vi "RebuildCmdListing.vi"(3 "Numeric":dbl, 4 "Contents":string, 5 "Params":T1(array[cluster]), 6 "String in":string) -> (1 "array":string[](array[string]), 2 "String out":string)   [LabVIEW 2012]
panel:
  out "Array":dbl[](array[numeric])
  out "Contents 2":string
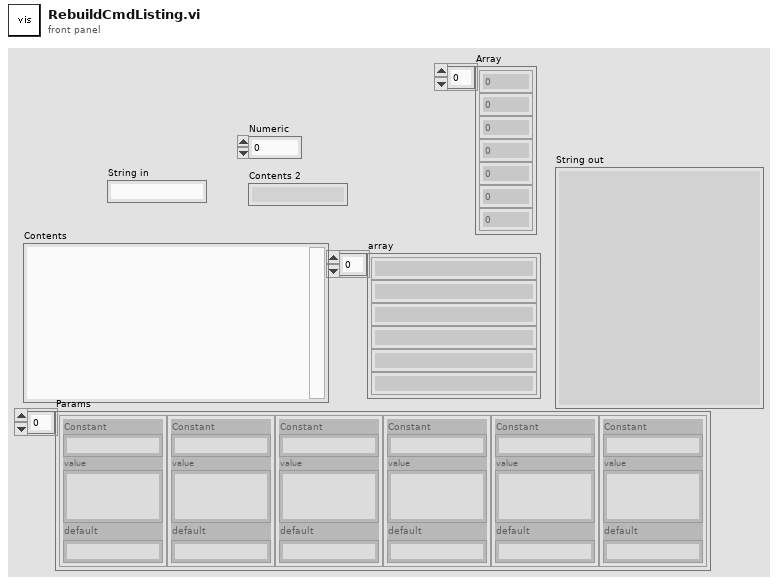
[diagram p1: front panel]
types:
  T1 = cluster{"Constant":string, "value":string, "default":string}[]
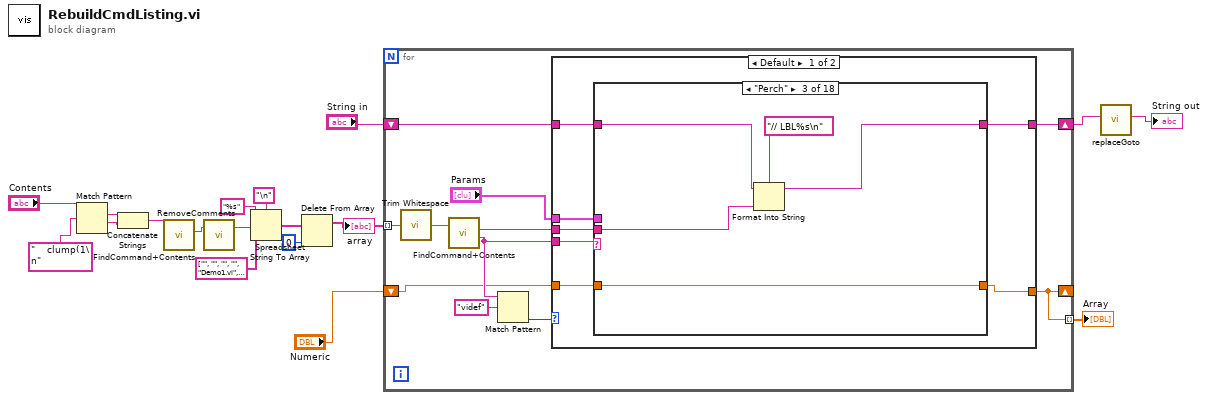
[diagram p0: block diagram]
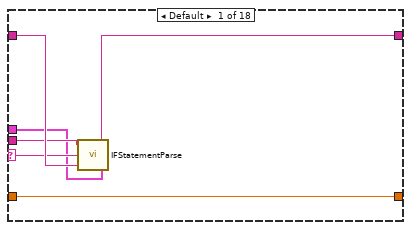
[diagram p2: hidden frame]
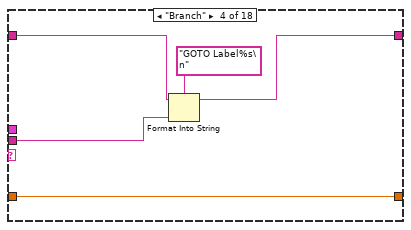
[diagram p4: hidden frame]
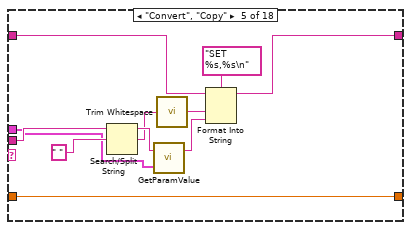
[diagram p5: hidden frame]
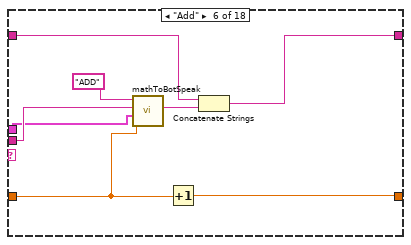
[diagram p6: hidden frame]
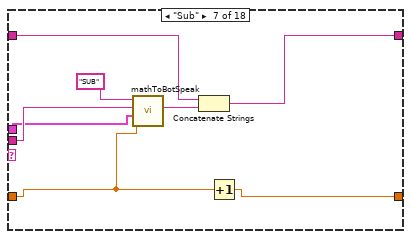
[diagram p7: hidden frame]
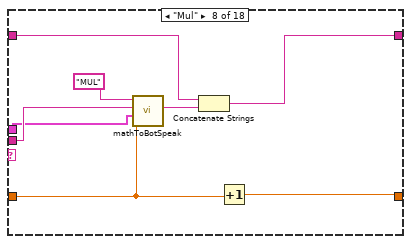
[diagram p8: hidden frame]
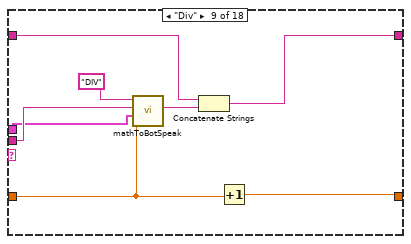
[diagram p9: hidden frame]
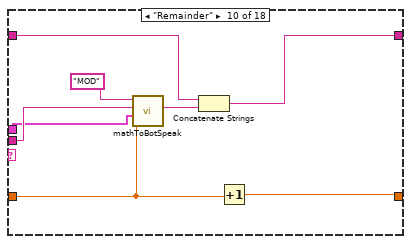
[diagram p10: hidden frame]
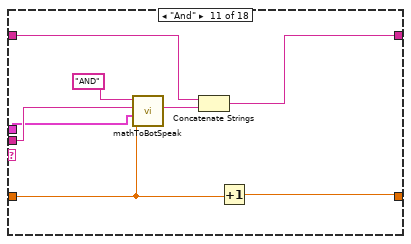
[diagram p11: hidden frame]
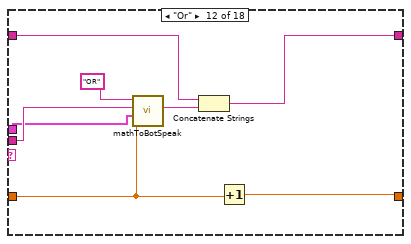
[diagram p12: hidden frame]
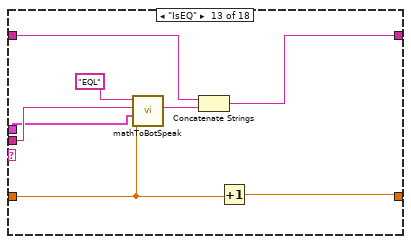
[diagram p13: hidden frame]
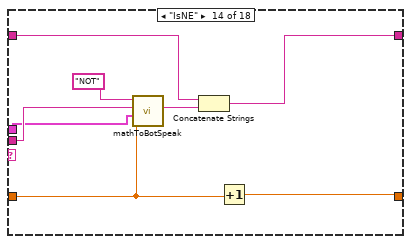
[diagram p14: hidden frame]
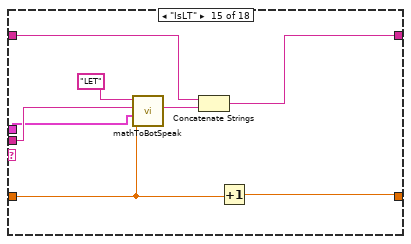
[diagram p15: hidden frame]
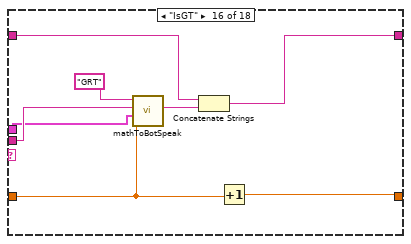
[diagram p16: hidden frame]
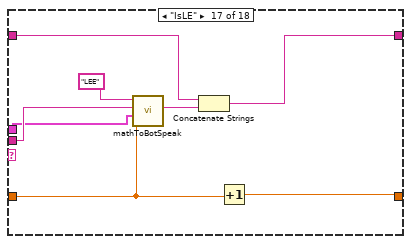
[diagram p17: hidden frame]
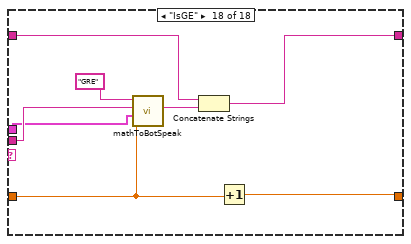
[diagram p18: hidden frame]
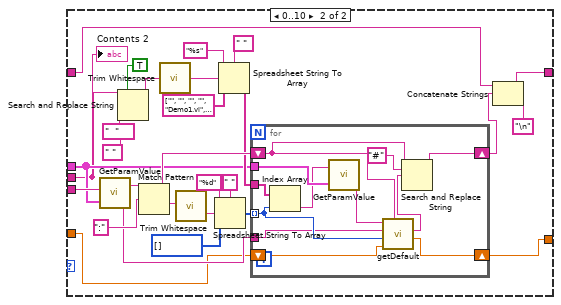
[diagram p19: hidden frame]
diagram:
  n1 = Match Pattern(string="Contents", regular expression="    clump(1\n") -> (match substring=w10:string, after substring=w11:string)  [unwired: 1 in, 2 out]
  n2 = Concatenate Strings(w10, w11) -> (w12:string)
  n3 = call <userlib>:"FindCommand+Contents.vi"("Via file in"=w12) -> ("Contents"=w13:string)  [unwired: 1 in, 3 out]
  n4 = call <userlib>:"RemoveComments.vi"("Via file in"=w13) -> ("Via file out"=w14:string)  [unwired: 2 in]
  n5 = Spreadsheet String To Array(delimiter (Tab)="\n", format string="%s", spreadsheet string=w14, array type (2D Dbl)=string[] ["", "", "", "", "Demo1.vi", "DigitalWrite.vi", "VS_Wait.vi", ""] ("Array 3")) -> (array=w17:string[])
  n6 = Delete From Array(array=w17, index=0) -> (array with subset deleted=w6:string[])  [unwired: 1 in, 1 out]
  "array" <- w6
  n7 = for {
    tunnel: w6 -> [w29] mode=indexing
    shift-right: [w26] -> w4
    shift-left: "String in" -> [w27]
    shift-right: [w19] -> _
    shift-left: "Numeric" -> [w20]
    tunnel: [w19] -> w2 mode=indexing
    n8 = call <vilib>:"Trim Whitespace.vi"("string"=w29) -> ("trimmed string"=w28:string)  [unwired: 1 in]
    n9 = call <userlib>:"FindCommand+Contents.vi"("Via file in"=w28) -> ("Contents"=w24:string, "command"=w23:string)  [unwired: 1 in, 2 out]
    n10 = Match Pattern(string=w23, regular expression="videf") -> (offset past match=w21:i32)  [unwired: 1 in, 3 out]
    n11 = case shown="Default" w21 {
      tunnel: w23 -> [w36 w197]
      tunnel: w27 -> [w35 w184]
      tunnel: [w33 w183] -> w26
      tunnel: "Params" -> [w32 w180]
      tunnel: w24 -> [w34 w177]
      tunnel: w20 -> [w31 w171]
      tunnel: [w30 w170] -> w19
      frame Default {
        n12 = case shown="\"Perch\"" w36 {
          selector: w36 -> [w40 _ _ _ _ _ _ _ _ _ _ _ _ _ _ _ _ _]
          tunnel: w35 -> [w42 w44 w48 w53 w64 w69 w77 w85 w93 w101 w109 w117 w125 w133 w141 w149 w157 w165]
          tunnel: w34 -> [w41 _ w47 w52 w62 w72 w80 w88 w96 w104 w112 w120 w128 w136 w144 w152 w160 w168]
          tunnel: [w39 w44 w46 w51 w57 w68 w76 w84 w92 w100 w108 w116 w124 w132 w140 w148 w156 w164] -> w33
          tunnel: w32 -> [w38 _ _ _ w61 w71 w79 w87 w95 w103 w111 w119 w127 w135 w143 w151 w159 w167]
          tunnel: [w37 w43 w45 w50 w59 w67 w75 w83 w91 w99 w107 w115 w123 w131 w139 w147 w155 w163] -> w30
          tunnel: w31 -> [w37 w43 w45 w50 w59 w66 w74 w82 w90 w98 w106 w114 w122 w130 w138 w146 w154 w162]
          frame Default {
            n13 = call <userlib>:"IFStatementParse.vi"("Params"=w38, "BotSpeak in"=w42, "Command"=w40, "Contents"=w41) -> ("BotSpeak out"=w39:string)  [unwired: 1 in]
          }
          frame "" {
          }
          frame "Perch" {
            n14 = Format Into String(format string="// LBL%s\n", initial string=w48, w47) -> (resulting string=w46:string)  [unwired: 1 in, 1 out]
          }
          frame "Branch" {
            n15 = Format Into String(format string="GOTO Label%s\n", initial string=w53, w52) -> (resulting string=w51:string)  [unwired: 1 in, 1 out]
          }
          frame "Convert", "Copy" {
            n16 = Search/Split String(string=w62, search string/char (-)=" ") -> (substring before match=w60:string, match + rest of string=w56:string)  [unwired: 1 in, 1 out]
            n17 = call <userlib>:"GetParamValue.vi"("Params"=w61, "command"=w60) -> ("value"=w58:string)  [unwired: 1 out]
            n18 = call <vilib>:"Trim Whitespace.vi"("string"=w56) -> ("trimmed string"=w55:string)  [unwired: 1 in]
            n19 = Format Into String(format string="SET %s,%s\n", initial string=w64, w55, w58) -> (resulting string=w57:string)  [unwired: 1 in, 1 out]
          }
          frame "Add" {
            n20 = call <userlib>:"mathToBotSpeak.vi"("Numeric"=w66, "Params"=w71, "String in"=w72, "Command"="ADD") -> ("resulting string"=w70:string)  [unwired: 7 in]
            n21 = Increment(x=w66) -> (x+1=w67:dbl)
            n22 = Concatenate Strings(w69, w70) -> (w68:string)
          }
          frame "Sub" {
            n23 = call <userlib>:"mathToBotSpeak.vi"("Numeric"=w74, "Params"=w79, "String in"=w80, "Command"="SUB") -> ("resulting string"=w78:string)  [unwired: 7 in]
            n24 = Concatenate Strings(w77, w78) -> (w76:string)
            n25 = Increment(x=w74) -> (x+1=w75:dbl)
          }
          frame "Mul" {
            n26 = call <userlib>:"mathToBotSpeak.vi"("Numeric"=w82, "Params"=w87, "String in"=w88, "Command"="MUL") -> ("resulting string"=w86:string)  [unwired: 7 in]
            n27 = Concatenate Strings(w85, w86) -> (w84:string)
            n28 = Increment(x=w82) -> (x+1=w83:dbl)
          }
          frame "Div" {
            n29 = call <userlib>:"mathToBotSpeak.vi"("Numeric"=w90, "Params"=w95, "String in"=w96, "Command"="DIV") -> ("resulting string"=w94:string)  [unwired: 7 in]
            n30 = Concatenate Strings(w93, w94) -> (w92:string)
            n31 = Increment(x=w90) -> (x+1=w91:dbl)
          }
          frame "Remainder" {
            n32 = call <userlib>:"mathToBotSpeak.vi"("Numeric"=w98, "Params"=w103, "String in"=w104, "Command"="MOD") -> ("resulting string"=w102:string)  [unwired: 7 in]
            n33 = Concatenate Strings(w101, w102) -> (w100:string)
            n34 = Increment(x=w98) -> (x+1=w99:dbl)
          }
          frame "And" {
            n35 = call <userlib>:"mathToBotSpeak.vi"("Numeric"=w106, "Params"=w111, "String in"=w112, "Command"="AND") -> ("resulting string"=w110:string)  [unwired: 7 in]
            n36 = Concatenate Strings(w109, w110) -> (w108:string)
            n37 = Increment(x=w106) -> (x+1=w107:dbl)
          }
          frame "Or" {
            n38 = call <userlib>:"mathToBotSpeak.vi"("Numeric"=w114, "Params"=w119, "String in"=w120, "Command"="OR") -> ("resulting string"=w118:string)  [unwired: 7 in]
            n39 = Concatenate Strings(w117, w118) -> (w116:string)
            n40 = Increment(x=w114) -> (x+1=w115:dbl)
          }
          frame "IsEQ" {
            n41 = call <userlib>:"mathToBotSpeak.vi"("Numeric"=w122, "Params"=w127, "String in"=w128, "Command"="EQL") -> ("resulting string"=w126:string)  [unwired: 7 in]
            n42 = Concatenate Strings(w125, w126) -> (w124:string)
            n43 = Increment(x=w122) -> (x+1=w123:dbl)
          }
          frame "IsNE" {
            n44 = call <userlib>:"mathToBotSpeak.vi"("Numeric"=w130, "Params"=w135, "String in"=w136, "Command"="NOT") -> ("resulting string"=w134:string)  [unwired: 7 in]
            n45 = Concatenate Strings(w133, w134) -> (w132:string)
            n46 = Increment(x=w130) -> (x+1=w131:dbl)
          }
          frame "IsLT" {
            n47 = call <userlib>:"mathToBotSpeak.vi"("Numeric"=w138, "Params"=w143, "String in"=w144, "Command"="LET") -> ("resulting string"=w142:string)  [unwired: 7 in]
            n48 = Concatenate Strings(w141, w142) -> (w140:string)
            n49 = Increment(x=w138) -> (x+1=w139:dbl)
          }
          frame "IsGT" {
            n50 = call <userlib>:"mathToBotSpeak.vi"("Numeric"=w146, "Params"=w151, "String in"=w152, "Command"="GRT") -> ("resulting string"=w150:string)  [unwired: 7 in]
            n51 = Concatenate Strings(w149, w150) -> (w148:string)
            n52 = Increment(x=w146) -> (x+1=w147:dbl)
          }
          frame "IsLE" {
            n53 = call <userlib>:"mathToBotSpeak.vi"("Numeric"=w154, "Params"=w159, "String in"=w160, "Command"="LEE") -> ("resulting string"=w158:string)  [unwired: 7 in]
            n54 = Concatenate Strings(w157, w158) -> (w156:string)
            n55 = Increment(x=w154) -> (x+1=w155:dbl)
          }
          frame "IsGE" {
            n56 = call <userlib>:"mathToBotSpeak.vi"("Numeric"=w162, "Params"=w167, "String in"=w168, "Command"="GRE") -> ("resulting string"=w166:string)  [unwired: 7 in]
            n57 = Concatenate Strings(w165, w166) -> (w164:string)
            n58 = Increment(x=w162) -> (x+1=w163:dbl)
          }
        }
      }
      frame 0..10 {
        n59 = call <userlib>:"GetParamValue.vi"("Params"=w180, "command"=w197) -> ("default"=w172:string, "value"=w196:string)
        n60 = Search and Replace String(replace all?=TRUE ("replace all? (F)"), input string=w177, search string="  ", replace string=" " ("replace string (\"\")")) -> (result string=w173:string)  [unwired: 4 in, 3 out]
        n61 = Match Pattern(string=w196, regular expression=":") -> (before substring=w187:string, after substring=w194:string)  [unwired: 1 in, 2 out]
        n62 = call <vilib>:"Trim Whitespace.vi"("string"=w173) -> ("trimmed string"=w178:string)  [unwired: 1 in]
        n63 = call <vilib>:"Trim Whitespace.vi"("string"=w194) -> ("trimmed string"=w179:string)  [unwired: 1 in]
        n64 = Spreadsheet String To Array(delimiter (Tab)=" ", format string="%d", spreadsheet string=w179, array type (2D Dbl)=i32[] [] ("Array 3")) -> (array=w185:i32[])
        n65 = Spreadsheet String To Array(delimiter (Tab)=" ", format string="%s", spreadsheet string=w178, array type (2D Dbl)=string[] ["", "", "", "", "Demo1.vi", "DigitalWrite.vi", "VS_Wait.vi", ""] ("Array 3")) -> (array=w186:string[])
        n66 = for {
          shift-right: [w209] -> w182
          shift-left: w187 -> [w198]
          tunnel: w186 -> [w207]
          tunnel: w185 -> [w202] mode=indexing
          tunnel: w180 -> [w206]
          tunnel: w172 -> [w201]
          shift-right: [w199] -> w170
          shift-left: w171 -> [w200]
          n67 = Index Array(array=w207, index=w202) -> (element=w205:string)
          n68 = call <userlib>:"GetParamValue.vi"("Params"=w206, "command"=w205) -> ("value"=w203:string)  [unwired: 1 out]
          n69 = call <userlib>:"getDefault.vi"("String"=w198, "var number"=w200, "location"=w202, "defaults"=w201, "value"=w203) -> ("var number 2"=w199:dbl, "value 2"=w204:string)  [unwired: 5 in]
          n70 = Search and Replace String(input string=w198, search string="#", replace string=w204) -> (result string=w209:string)  [unwired: 5 in, 3 out]
        }
        n71 = Concatenate Strings(w184, w182, "\n" ("delimiter (Tab)")) -> (w183:string)
        "Contents 2" <- w177
      }
    }
  }
  "Array" <- w2
  n72 = call <userlib>:"replaceGoto.vi"("String in"=w4) -> ("BotSpeak Out"=→"String out":string)  [unwired: 10 in]
